vi "Status.vi"() -> (2 "Schritt Status":string, 3 "Statusarray":string[](array[string]))   [LabVIEW 2019]
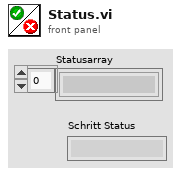
[diagram p1: front panel]
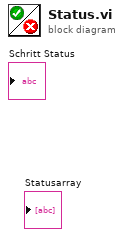
[diagram p0: block diagram]
diagram:
